vi "CopySourceFiles.vi"(4 "Folder to Exclude":string[](array[string])=[".git", "examples"], 6 "File Types":string[](array[string])=["*.h", "*.cpp", "*.c", "*.ino"], 8 "Error In":errorcluster, 10 "Destination Path":path, 11 "Source Path":path) -> (0 "Error Out":errorcluster)   [LabVIEW 2010]
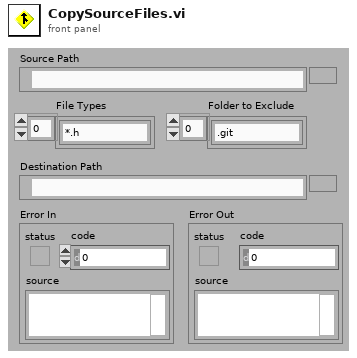
[diagram p1: front panel]
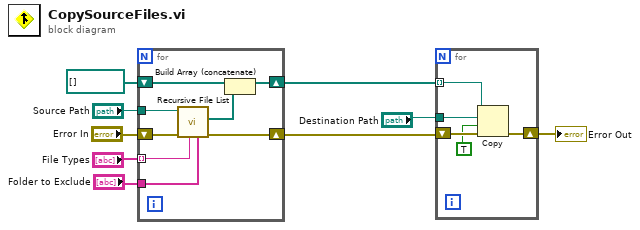
[diagram p0: block diagram]
diagram:
  n1 = for {
    tunnel: "Source Path" -> [w16]
    shift-right: [w13] -> w6
    shift-left: "Error In" -> [w17]
    tunnel: "File Types" -> [w15] mode=indexing
    tunnel: "Folder to Exclude" -> [w14]
    shift-right: [w11] -> w4
    shift-left: path[] [] ("All Files in Dir") -> [w12]
    n2 = call <vilib>:"Recursive File List.vi"("Folders to Exclude"=w14, "pattern"=w15, "error in (no error)"=w17, "Folder Path"=w16) -> ("error out"=w13:errorcluster, "All Files in Dir"=w10:path[])  [unwired: 3 in, 3 out]
    n3 = Build Array (concatenate)(w12, w10) -> (w11:path[])
  }
  n4 = for {
    shift-right: [w21] -> w3
    shift-left: w6 -> [w22]
    tunnel: "Destination Path" -> [w20]
    tunnel: w4 -> [w19] mode=indexing
    n5 = Copy(8:w22, 9:TRUE ("overwrite (F)"), 10:w20, 11:w19) -> (0:w21:errorcluster)  [unwired: 1 in, 2 out]
  }
  "Error Out" <- w3
